vi "histogram.vi"(7 "# bins":i32=20, 10 "img":u16[][](array[numeric])) -> (2 "histogram":cluster{"Axis":dbl[], "Histogram":i32[]}(graph))   [LabVIEW 2020]
uses:
  <vilib>/Analysis/NI_AALPro.lvlib
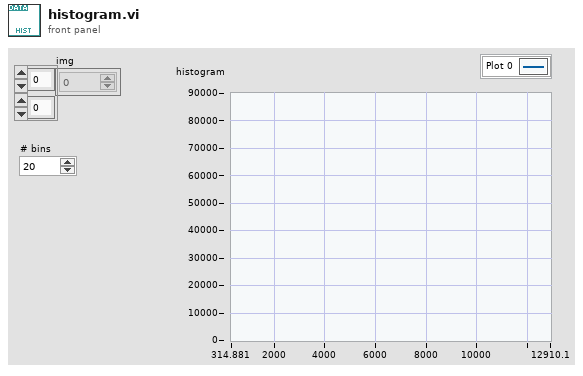
[diagram p1: front panel]
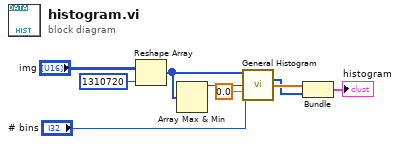
[diagram p0: block diagram]
diagram:
  n1 = Reshape Array("img", 1310720 ("dimension size")) -> (w4:u16[])
  n2 = Array Max & Min(array=w4) -> (max value=w3:u16)  [unwired: 3 out]
  n3 = call <vilib>:"General Histogram.vi"("X"=w4, "max"=w3, "min"=0.0, "# bins"="# bins") -> ("Histogram"=w2:i32[], "Axis"=w7:dbl[])  [unwired: 7 in, 3 out]
  n4 = Bundle("Axis"=w7, "Histogram"=w2) -> (→"histogram":cluster{"Axis":dbl[], "Histogram":i32[]})  [unwired: 1 in]
